vi "NAI8810A.vi"(8 "error in":errorcluster) -> (0 "error out":errorcluster)   [LabVIEW 2020]
uses:
  SubVIs/NAI8810A_TypeDefs.llb/AngleDifferenceButton.ctl
  <vilib>/Utility/miscctls.llb/LVPointTypeDef.ctl
  LabVIEW 2020 Toolkits/toolkits_lv2020_32bit/Synchronization.llb/SynchRefs_SetGet.ctl
  SubVIs/NAI8810A_TypeDefs.llb/NAI8810A_Command.ctl
  LabVIEW 2020 Toolkits/VI Server Toolkit/VI Server Libraries/VI Server_GetControl.llb/VI Server_STR_Get.vi
  <vilib>/Utility/inputDevices.llb/closeKeyboard.vi
  LabVIEW 2020 Toolkits/VI Server Toolkit/VI Server Toolkit LV2013.lvlib
panel:
  out "System.Message":string
  in  "UDP.Setup":bool
  in  "Help":bool
  in  "FP.Hide":bool caption="FrontPanel.Hide"
  in  "EXIT":bool
  in  "Tab.Main":T1(tab)
  in  "Ch1.Hold":bool
  in  "Tab.Ch1.Help":bool
  in  "Tab.Ch1.SetUp":bool
  in  "Tab.Ch1.IntRef":bool
  in  "Tab.Ch1.DualCh":bool
  in  "Tab.Ch1.Ch2":bool
  in  "Tab.Ch1.Ch1":bool
  out "Ch1.Degree":dbl caption="Degree" format="%0.4f"
  in  "Ch1.Input.Front/Rear":bool
  in  "Ch1.Local/Remote":bool
  in  "Ch1.Ratio":bool
  in  "Ch1.Graph":bool
  in  "Ch1.AnalogDisplay":bool
  in  "Ch1.EnableAngleOffsetCalc":bool
  in  "Ch1.TestAngleReadings":bool
  in  "Ch1.Ave.AnglesReadings":bool
  in  "Ch1.SYN/RSL":bool
  in  "Ch1.Internal/External.Ref":bool
  out "Ch1.Velocity":dbl format="%0.1f dps"
  out "Ch1.Frequency":dbl format="%0.2f Hz"
  out "Ch1.Line-to-Line.Voltage":dbl format="%0.2f mV"
  out "Ch1.Ref.Voltage":dbl format="%0.2f mV"
  in  "Ch2.Ave.AnglesReadings":bool
  in  "Ch2.Input.Front/Rear":bool
  out "Ch2.Line-to-Line.Voltage":dbl format="%0.2f mV"
  in  "Ch2.Hold":bool
  in  "Ch2.Graph":bool
  in  "Ch2.SYN/RSL":bool
  in  "Ch2.Internal/External.Ref":bool
  in  "Ch2.EnableAngleOffsetCalc":bool
  in  "Ch2.TestAngleReadings":bool
  in  "Ch2.Ratio":bool
  in  "Ch2.Local/Remote":bool
  out "Ch2.Velocity":dbl format="%0.1f dps"
  out "Ch2.Ref.Voltage":dbl format="%0.2f mV"
  out "Ch2.Degree":dbl caption="Degree" format="%0.4f"
  in  "Tab.Ch2.Ch2":bool
  in  "Tab.Ch2.Ch1":bool
  in  "Tab.Ch2.DualCh":bool
  in  "Tab.Ch2.IntRef":bool
  in  "Tab.Ch2.SetUp":bool
  in  "Tab.Ch2.Help":bool
  out "Ch2.Frequency":dbl format="%0.2f Hz"
  in  "Ch2.AnalogDisplay":bool
  in  "Ch1-2.Local/Remote":bool
  in  "Ch1-2.Ch2.AngleDifference":T2
  out "Ch1-2.Ch2.Frequency":dbl format="%0.2f Hz"
  out "Ch1-2.Ch2.Line-to-Line.Voltage":dbl format="%0.2f mV"
  out "Ch1-2.Ch2.Ref.Voltage":dbl format="%0.2f mV"
  in  "Ch1-2.Ch2.Ave.AnglesReadings":bool
  in  "Ch1-2.Ch2.Hold":bool
  in  "Ch1-2.Ch2.SYN/RSL":bool
  in  "Ch1-2.Ch2.Internal/External.Ref":bool
  out "Ch1-2.Ch2.Degree":dbl caption="Degree" format="%0.4f"
  in  "Ch1-2.Ch1.TestAngleReadings":bool
  in  "Ch1-2.Ch1.Ave.AnglesReadings":bool
  out "Ch1-2.Ch1.Line-to-Line.Voltage":dbl format="%0.2f mV"
  out "Ch1-2.Ch1.Ref.Voltage":dbl format="%0.2f mV"
  out "Ch1-2.Ch1.Frequency":dbl format="%0.2f Hz"
  in  "Ch1-2.Graph":bool
  in  "Ch1-2.Ratio":bool
  in  "Ch1-2.Input.Front/Rear":bool
  in  "Ch1-2.Ch1.SYN/RSL":bool
  in  "Ch1-2.Ch1.Internal/External.Ref":bool
  in  "Ch1-2.Ch1.Hold":bool
  out "Ch1-2.Ch1.Degree":dbl caption="Degree" format="%0.4f"
  in  "Tab.Ch1-2.SetUp":bool
  in  "Tab.Ch1-2.IntRef":bool
  in  "Tab.Ch1-2.Ch2":bool
  in  "Tab.Ch1-2.Ch1":bool
  in  "Tab.Ch1-2.Ch1-2":bool
  in  "Tab.Ch1-2.Help":bool
  in  "Ch1-2.Ch2.TestAngleReadings":bool
  in  "InternalRef.Frequency.Increment":bool
  in  "InternalRef.Input.Front/Rear":bool
  in  "InternalRef.Delta":u16=1 min=1 max=20000
  in  "InternalRef.115V":bool
  in  "InternalRef.26V":bool
  in  "InternalRef.Signal.Out":u16(ring) items=["AVAILABLE", "NOT AVAILABLE"]
  in  "InternalRef.Local/Remote":bool
  in  "InternalRef.Ratio":bool
  in  "InternalRef.Graph":bool
  in  "InternalRef.Frequency":dbl=47.0 caption="Degree" min=47.0 max=20000.0 step=0.1 format="%0.2f"
  in  "InternalRef.Voltage":dbl=2.0 caption="Degree" min=2.0 max=115.0 step=0.1 format="%0.1f"
  in  "Tab.IntRef.Help":bool
  in  "Tab.IntRef.IntRef":bool
  in  "Tab.IntRef.Ch1":bool
  in  "Tab.IntRef.Ch2":bool
  in  "Tab.IntRef.Ch1-2":bool
  in  "Tab.IntRef.SetUp":bool
  in  "AutomaticUpdate":bool caption="Automatic Update"
  in  "TCP/IP.Setup":bool
  in  "Ch2.Bandwidth.Value":u16=6 caption="Bandwidth Value (6-1200 Hz)" min=6 max=1200 format="%d Hz"
  in  "Ch2.AutoBandwidth":bool caption="Auto-Bandwidth"
  in  "Ch1.Bandwidth.Value":u16=6 caption="Bandwidth Value (6-1200 Hz)" min=6 max=1200 format="%d Hz"
  in  "Ch1.AutoBandwidth":bool caption="Auto-Bandwidth"
  in  "AngleResolution":u16(ring) caption="Angle Res:" items=["0", "1", "2", "3", "4"]
  in  "AngleDisplay.Format":u16(ring) caption="Angle Display:" items=["360", "180", "MIN"]
  in  "Setup.DONE":bool
  in  "UpdateTime.Ref.Parameters":u32=5 caption="Ref. Data" min=5 max=20000 format="%d msec"
  in  "UpdateTime.Degrees":u32=5 caption="Degrees" min=5 max=20000 format="%d msec"
  out "UDP.Responce.String":string caption="UDP: Responce String"
  in  "UDP.Responce.String.Monitor":bool
  in  "UDP.Test.String2.Send":bool
  in  "UDP.Test.String2":string caption="UDP: Test String 2"
  in  "UDP.IP.Address":string caption="UDP: IP Address"
  in  "UDP.LocalPort.Write":u16 caption="UDP: Local Port.Write"
  in  "UDP.Port.RT":u16 caption="UDP: Port.RT"
  in  "UDP.Port.BC":u16 caption="UDP: Port.BC"
  in  "UDP.Test.String1":string caption="UDP: Test String 1"
  in  "UDP.Test.String1.Send":bool
  in  "AveAnglesReadings.DONE":bool
  in  "Ch2.AveragingInterval":u16=10 caption="Averaging Interval" min=10 max=10000 format="%d msec"
  in  "Ch2.AverageAnglesReadings":bool caption="Ch2: Average Angles Readings"
  in  "Ch1.AveragingInterval":u16=10 caption="Averaging Interval" min=10 max=10000 format="%d msec"
  in  "Ch1.AverageAnglesReadings":bool caption="Ch1: Average Angles Readings"
  in  "Ch2.TestAngleReading.Step":dbl=0.0001 caption="Angle Step" min=0.0001 max=359.9999 format="%0.4f deg"
  in  "Ch2.TestAngleReading.Limit.LO":dbl caption="Angle Limit LO" min=0.0 max=359.9999 format="%0.4f deg"
  in  "Ch2.TestAngleReading.Limit.HI":dbl caption="Angle Limit HI" min=0.0 max=359.9999 format="%0.4f deg"
  in  "Ch2.TestAngleReading.Comparision.Mode":bool caption="Ch1.TestAngleReading"
  in  "Ch2.TestAngleReading.ENBL":bool caption="Ch1.TestAngleReading"
  in  "Ch1.TestAngleReading.Step":dbl=0.0001 caption="Angle Step" min=0.0001 max=359.9999 format="%0.4f deg"
  in  "Ch1.TestAngleReading.Limit.LO":dbl caption="Angle Limit LO" min=0.0 max=359.9999 format="%0.4f deg"
  in  "Ch1.TestAngleReading.Limit.HI":dbl caption="Angle Limit HI" min=0.0 max=359.9999 format="%0.4f deg"
  in  "Ch1.TestAngleReading.Comparision.Mode":bool caption="Ch1.TestAngleReading"
  in  "Ch1.TestAngleReading.ENBL":bool caption="Ch1.TestAngleReading"
  in  "TestAnglesReadings.DONE":bool
  in  "Ratio.Value":u8=2 caption="Ratio                              : 1" min=1
  in  "Ratio.Mode":bool
  in  "Ratio.DONE":bool
  in  "Chart.Config.ClearBuffer":bool
  in  "Chart.Config":bool
  in  "Chart.Start":bool
  in  "Chart.DONE":bool
  out "Chart":dbl(graph)
  in  "Chart.Config.SamplingRate.Units":u16(ring) items=["msec", "sec", "min"]
  in  "Chart.Config.SamplingRate":u16 caption="Sampling Rate"
  in  "Chart.Config.DataToPlot":u16(ring) caption="Data To Plot" items=["Angle", "Angl Error", "Velocity"]
  in  "Chart.Config.ChannelSelection":u16(ring) caption="Chan Display" items=["BOTH", "CH1", "CH2"]
  in  "Chart.Config.DataToPlot.Step":dbl=0.0001 caption="Angle Step" min=0.0001 max=359.9999 format="%0.4f deg"
  in  "GraphConfig.DONE":bool
  in  "MonitorCommandExecution":bool caption="Monitor Command Execution"
  in  "TCP/IP.Command.Send":bool
  out "TCP/IP.InstrumentResponce":string caption="Instrument Responce"
  in  "TCP/IP.Command":string="*IDN?" caption="Command"
  in  "TCP/IP.Instrument.ID":string="NORTH ATLANTIC,5330A-10" caption="TCP/IP: Instrument ID"
  in  "TCP/IP.Port":u16=23 caption="TCP/IP: Port"
  in  "TCP/IP.Address":string="192.168.4.5" caption="TCP/IP: Address"
  in  "TCP/IP.DONE":bool
  # "Options: Current Configuration"
  # "Options: Bandwidth"
  # "Channel 2"
  # "Channel 1"
  # "Update Time"
  # "Chanel 2"
  # "Chanel 1"
  # "Ratio"
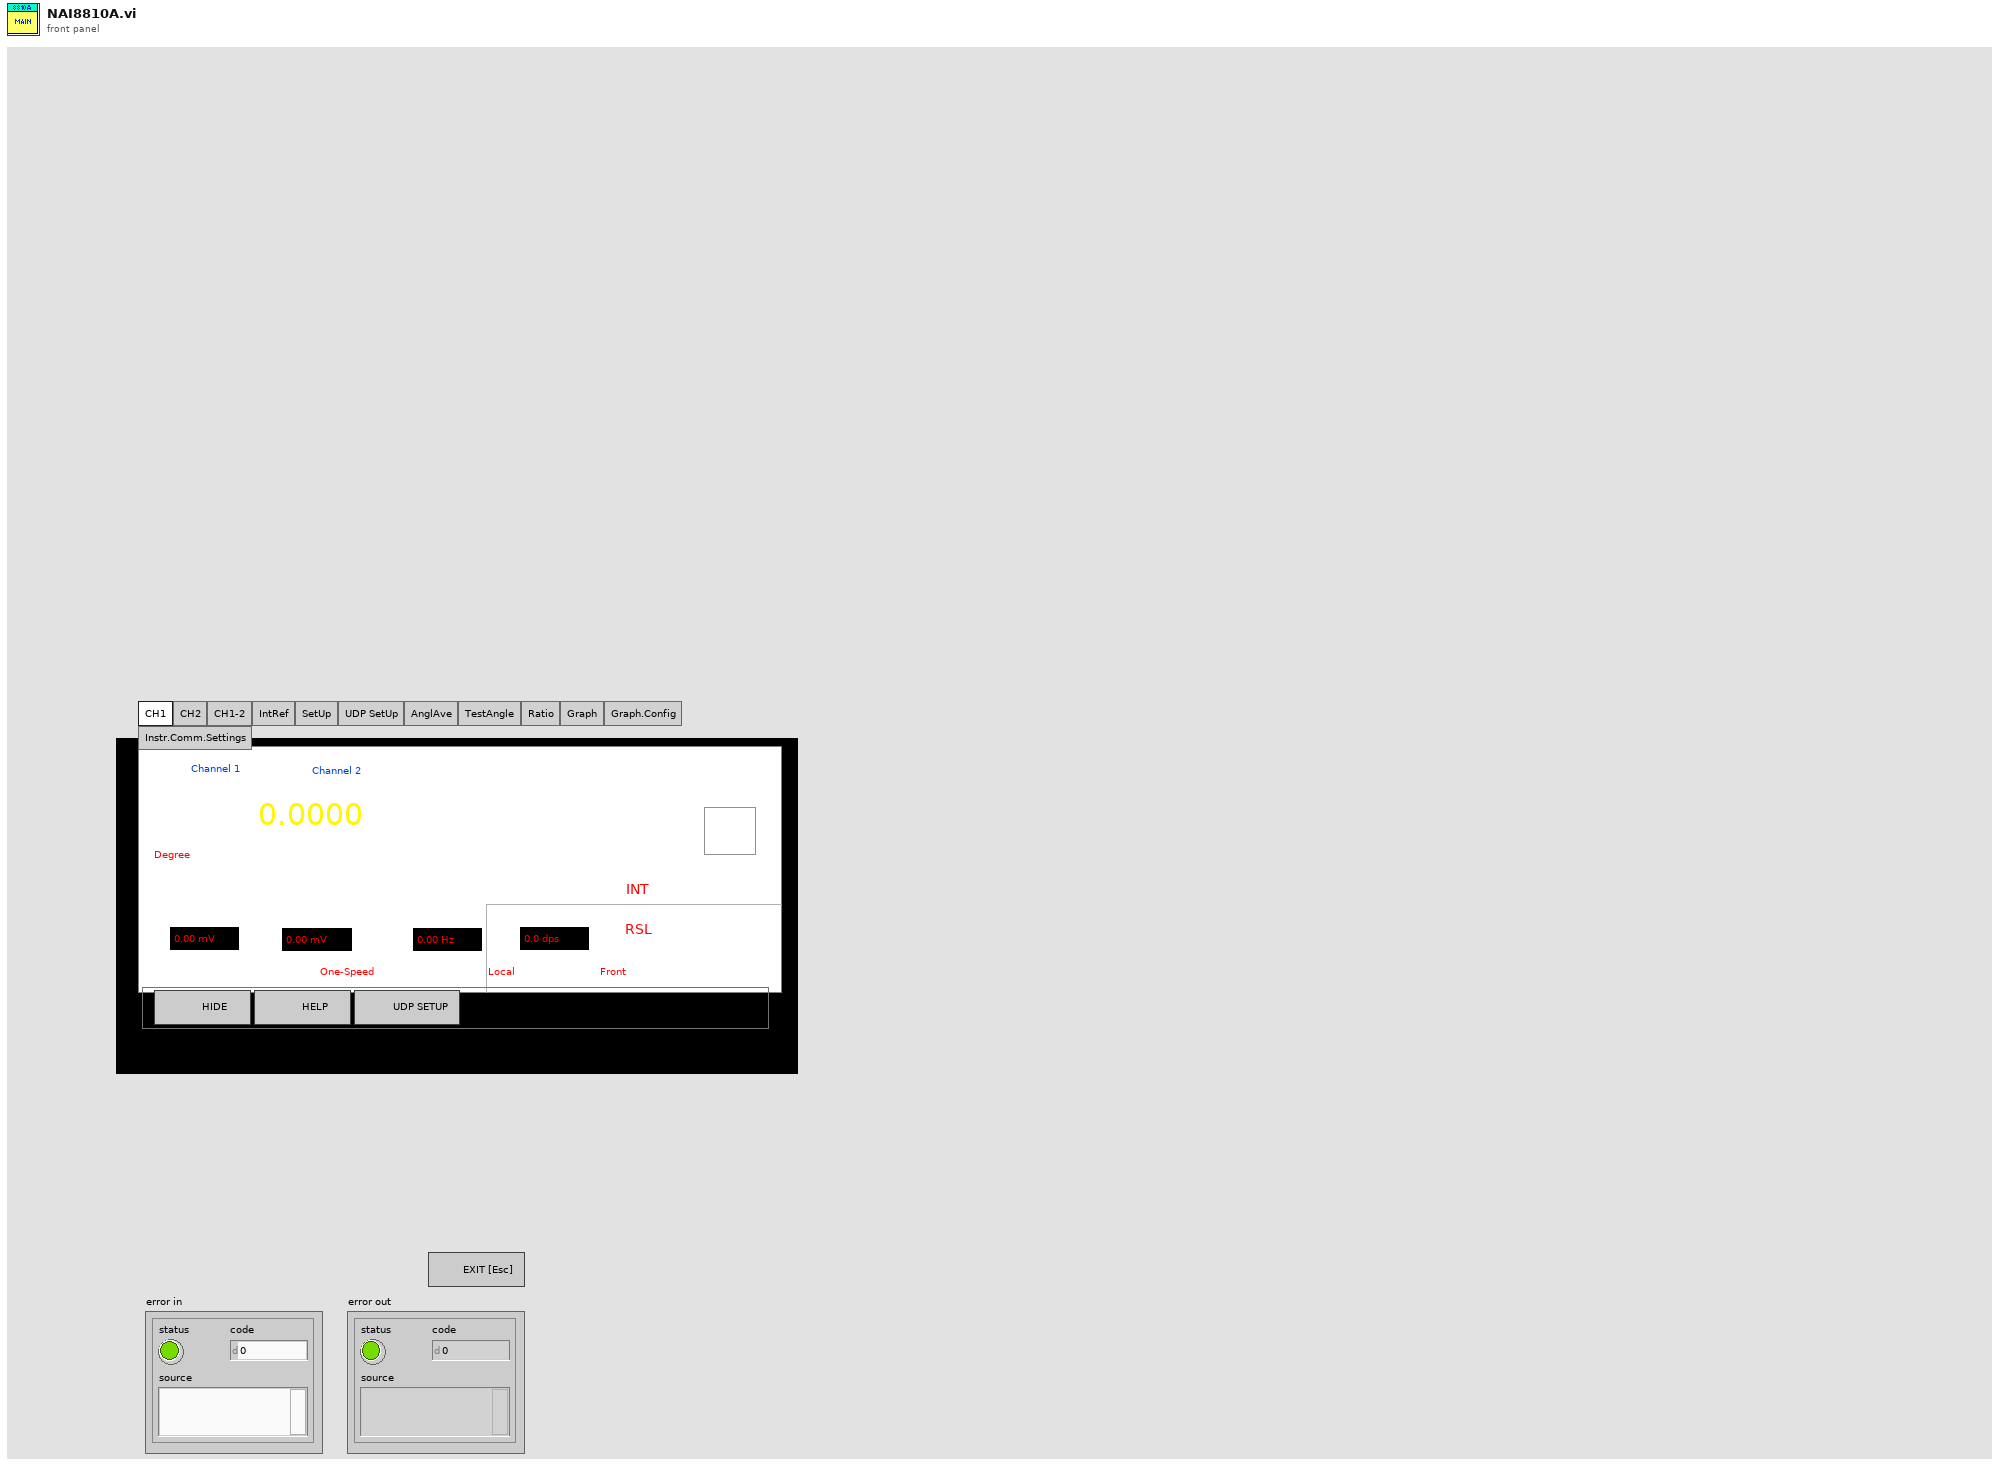
[diagram p1: front panel]
types:
  T1 = enum32{"CH1", "CH2", "CH1-2", "IntRef", "SetUp", "UDP SetUp", "AnglAve", "TestAngle", "Ratio", "Graph", "Graph.Config", "Instr.Comm.Settings"}
  T2 = typedef "AngleDifferenceButton.ctl" = bool
  T3 = typedef "LVPointTypeDef.ctl" = cluster{"Horizontal":i16, "Vertical":i16}
  T4 = typedef "VI Server_RefsCluster.ctl" = cluster{"Labels":string[], "Refs":refnum<vi>[], "VI Ref":refnum<vi>}
  T5 = typedef "SynchRefs_SetGet.ctl" = enum16{"Set", "Get"}
  T6 = typedef "NAI8810A_Command.ctl" = enum16{"", "*IDN?", "Reference Mode", "Signal Mode", "Channel 1 Input Connector", "Track/Latch Angle", "Reference Generator Voltage", "Reference Generator Frequency", "Reference Generator Output State", "Reference Generator Overcurrent State", "Reference Generator Overcurrent State RST ", "Angle Difference", "Angle Difference Get", "Angle Ch1", "Reference Voltage", "Angle Ch2", "Angle Ch1-2", "Angle Averaging ON/OFF", "Ch1.Angle Averaged", "Ch2.Angle Averaged", "Angle.AverageRate", "Ch1.Velocity", "Ch2.Velocity", "Ch1.Line-to-Line Voltage", "Ch2.Line-to-Line Voltage", "Ch1.ReferenceVoltage", "Ch2.ReferenceVoltage", "Ch1.ReferenceFrequency", "Ch2.ReferenceFrequency", "LOCAL/REMOTE", "ANG_LIMIT.ON|OFF", "ANG_LIMIT.CMP.ABS|ERR", "ANG_LIMIT.HI", "ANG_LIMIT.LO", "ANG_LIMIT.STEP", "Ratio", "AngleDisplay.Format", "Angles.Resolution", "Bandwidth.AUTO", "Bandwidth.SET", "Plot.ChannelSelection", "Data-to-Plot", "Buffering: SampleRate", "Clear Buffer", "Buffer: Record"}
  T7 = enum32{"CH1", "CH2", "CH1-2", "IntRef", "SetUp", "UDP SetUp", "AnglAve", "TestAngle"}
  T8 = enum32{"CH1", "CH2", "CH1-2", "IntRef", "SetUp", "UDP SetUp", "AnglAve", "TestAngle", "Ratio", "Graph", "Graph.Config"}
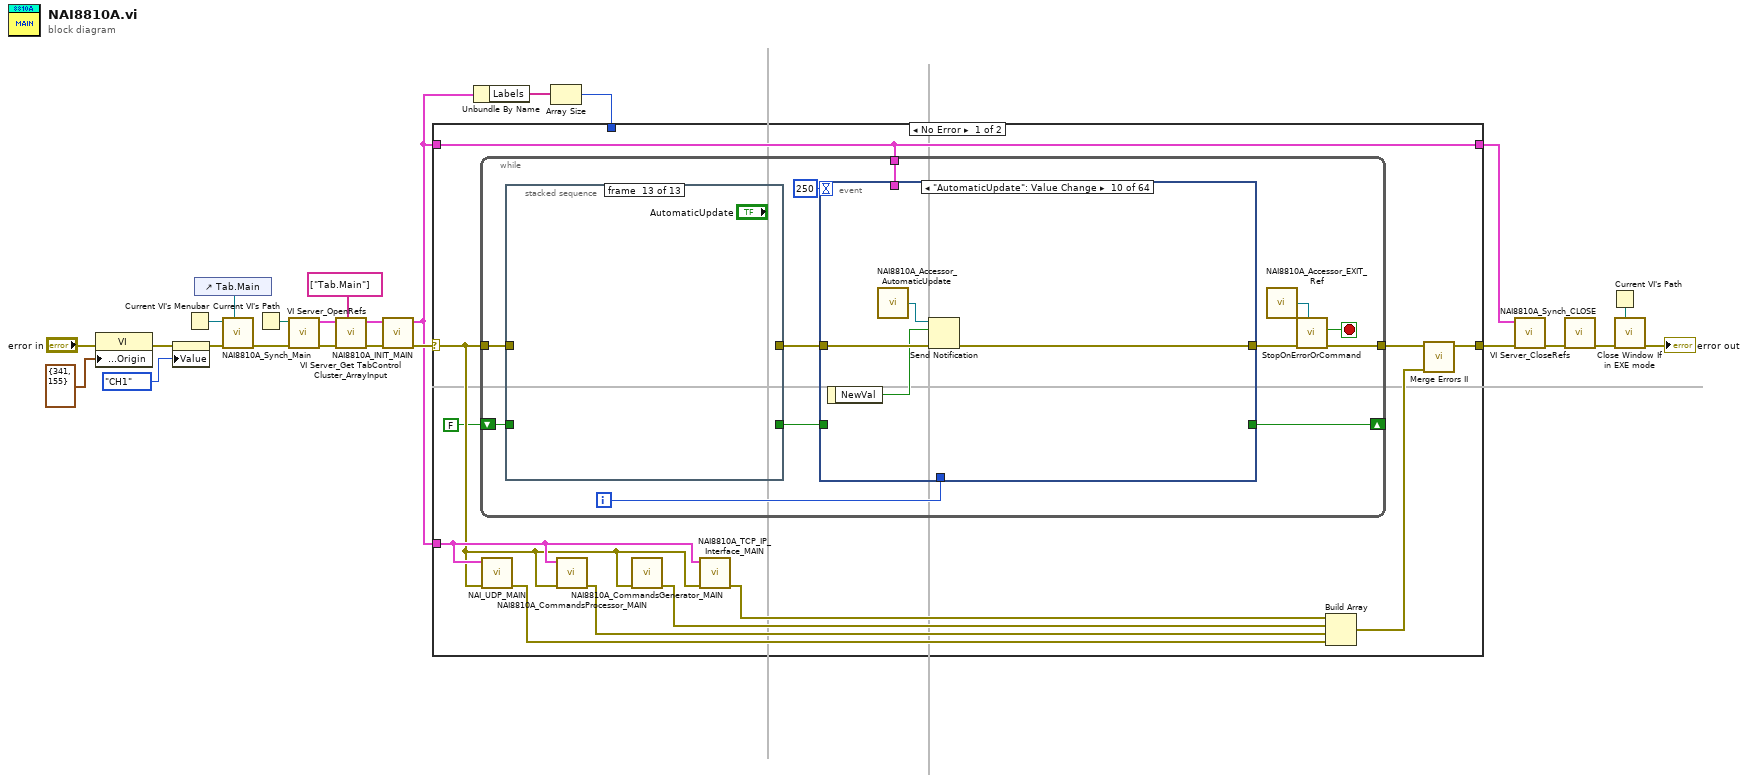
[diagram p0: block diagram]
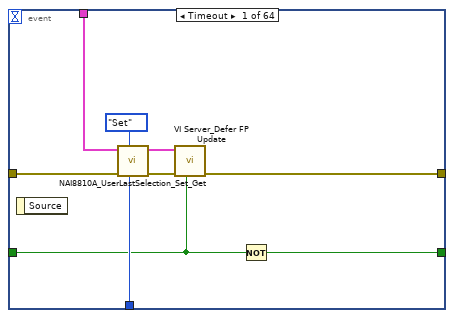
[diagram p2: hidden frame]
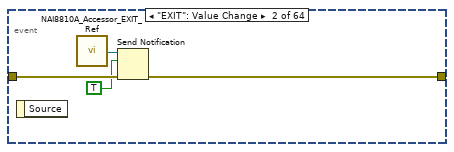
[diagram p3: hidden frame]
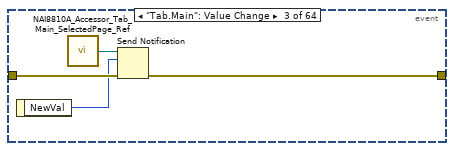
[diagram p4: hidden frame]
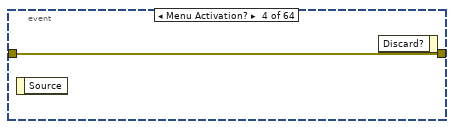
[diagram p5: hidden frame]
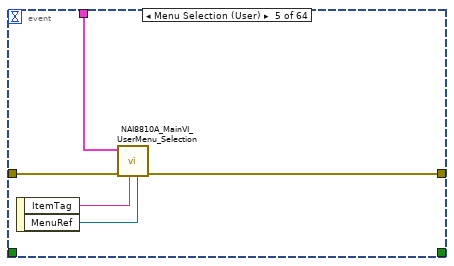
[diagram p6: hidden frame]
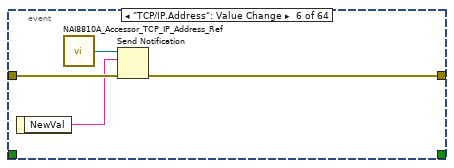
[diagram p7: hidden frame]
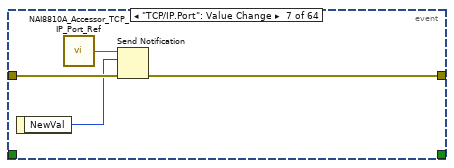
[diagram p8: hidden frame]
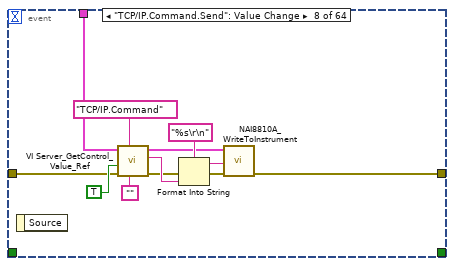
[diagram p9: hidden frame]
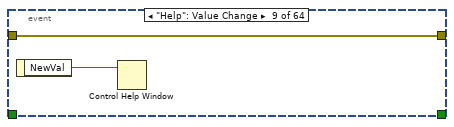
[diagram p10: hidden frame]
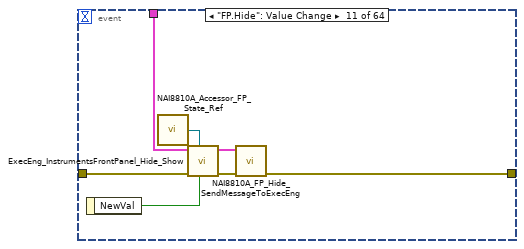
[diagram p11: hidden frame]
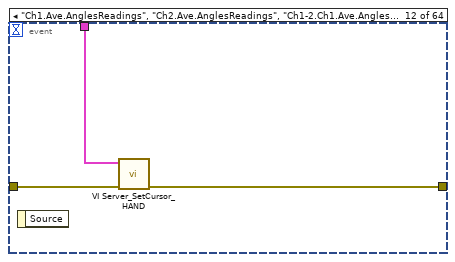
[diagram p12: hidden frame]
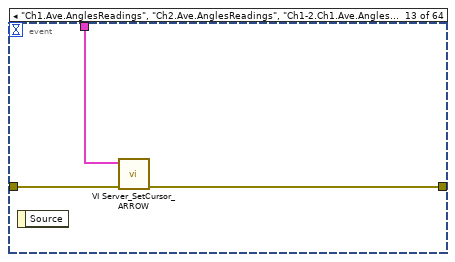
[diagram p13: hidden frame]
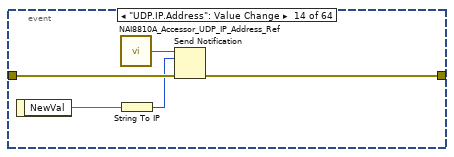
[diagram p14: hidden frame]
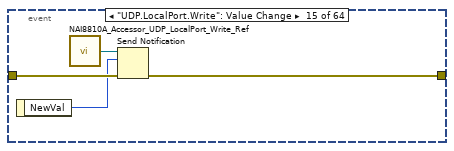
[diagram p15: hidden frame]
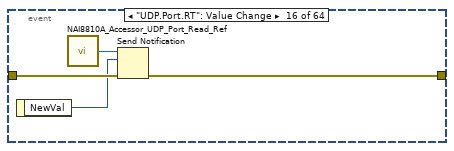
[diagram p16: hidden frame]
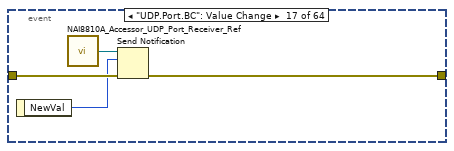
[diagram p17: hidden frame]
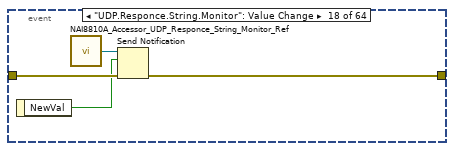
[diagram p18: hidden frame]
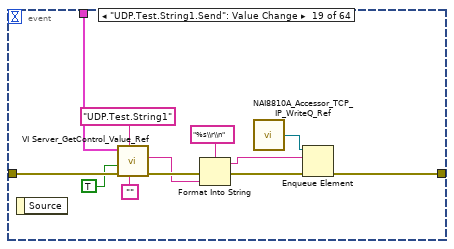
[diagram p19: hidden frame]
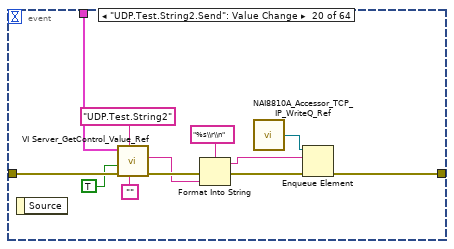
[diagram p20: hidden frame]
diagram:
  n1 = property class="VI"(error in="error in", "Front Panel Window:Origin"=T3 {"Horizontal"=341, "Vertical"=155}) -> (error out=w3:errorcluster)  [unwired: 1 in, 1 out]
  n2 = property on="Tab.Main" class="TabCtl (strict)"(error in=w3, "Value"=T1."CH1" ("Tab.Main")) -> (error out=w2:errorcluster)  [unwired: 1 in, 1 out]
  n3 = Current VI's Menubar() -> (w7:refnum<k9>)
  n4 = control-ref of="Tab.Main"() -> (w11:refnum<vi>)
  n5 = call "NAI8810A_Synch_Main.vi"("Tab.Main.Ref"=w11, "error in"=w2, "menu reference"=w7) -> ("error out"=w14:errorcluster)  [unwired: 8 in]
  n6 = Current VI's Path() -> (path=w21:path)
  n7 = call "VI Server_OpenRefs.vi"("error in"=w14, "VI Path"=w21) -> ("error out"=w24:errorcluster, "VI Server.RefsCluster"=w23:T4)  [unwired: 8 in]
  n8 = call "VI Server_Get TabControl Cluster_ArrayInput.vi"("TabControl Labels[]"=string[] ["Tab.Main"], "error in"=w24, "VI Server Cluster"=w23) -> ("error out"=w16:errorcluster, "VI Server Cluster.OUT"=w15:T4)  [unwired: 7 in]
  n9 = call "NAI8810A_INIT_MAIN.vi"("error in (no error)"=w16, "VI Server Cluster"=w15) -> ("error out"=w17:errorcluster, "VI Server Cluster DUP"=w10:T4)  [unwired: 8 in]
  n10 = Unbundle By Name(w10) -> ("Labels"=w9:string[])
  n11 = Array Size(array=w9) -> (size(s)=w8:i32)
  n12 = case shown="No Error" w17 {
    selector: w17 -> [w27 w434]
    tunnel: [w34 w434] -> w20
    tunnel: w10 -> [w28 _]
    tunnel: w10 -> [w31 w433]
    tunnel: [w31 w433] -> w18
    tunnel: w8 -> [_ _]
    frame No Error {
      n13 = while {
        tunnel: w27 -> [w47]
        tunnel: [w44] -> w35
        tunnel: w31 -> [w40]
        shift-right: [w36] -> _
        shift-left: FALSE -> [w38]
        i -> [w39]
        stop <- w42 stop-if-true
        n14 = stacked-sequence {
          tunnel: w47 -> [w431 _ _ _ _ _ _ _ _ _ _ _ _]
          tunnel: [w431 _ _ _ _ _ _ _ _ _ _ _ _] -> w45
          tunnel: w38 -> [_ w432 _ _ _ _ _ _ _ _ _ _ _]
          tunnel: [_ w432 _ _ _ _ _ _ _ _ _ _ _] -> w37
          frame #0 {
          }
          frame #1 {
          }
          frame #2 {
          }
          frame #3 {
          }
          frame #4 {
          }
          frame #5 {
          }
          frame #6 {
          }
          frame #7 {
          }
          frame #8 {
          }
          frame #9 {
          }
          frame #10 {
          }
          frame #11 {
          }
          frame #12 {
          }
        }
        n15 = event shown="[9] \"AutomaticUpdate\": Value Change" {
          selector: _ -> [_ _ _ _ _ _ _ _ _ _ _ _ _ _ _ _ _ _ _ _ _ _ _ _ _ _ _ _ _ _ _ _ _ _ _ _ _ _ _ _ _ _ _ _ _ _ _ _ _ _ _ _ _ _ _ _ _ _ _ _ _ _ _ _]
          dyn-events: _ -> [_ _ _ _ _ _ _ _ _ _ _ _ _ _ _ _ _ _ _ _ _ _ _ _ _ _ _ _ _ _ _ _ _ _ _ _ _ _ _ _ _ _ _ _ _ _ _ _ _ _ _ _ _ _ _ _ _ _ _ _ _ _ _ _]
          timeout: 250 -> [_ _ _ _ _ _ _ _ _ _ _ _ _ _ _ _ _ _ _ _ _ _ _ _ _ _ _ _ _ _ _ _ _ _ _ _ _ _ _ _ _ _ _ _ _ _ _ _ _ _ _ _ _ _ _ _ _ _ _ _ _ _ _ _]
          tunnel: w45 -> [w56 w60 w64 w65 w70 w74 w78 w84 w92 w96 w103 w106 w109 w114 w118 w122 w126 w130 w142 w154 w158 w160 w168 w183 w198 w213 w225 w228 w231 w239 w251 w258 w260 w264 w267 w269 w272 w277 w285 w293 w304 w315 w326 w333 w335 w339 w343 w346 w350 w354 w358 w371 w384 w387 w392 w395 w402 w405 w411 w417 w420 w423 w424 w430]
          tunnel: [w48 w58 w62 w65 w68 w73 w75 w79 w92 w95 w98 w104 w107 w113 w117 w121 w125 w127 w141 w153 w155 w163 w178 w193 w204 w219 w224 w227 w230 w240 w252 w259 w261 w262 w266 w268 w271 w278 w284 w289 w298 w309 w320 w332 w336 w337 w341 w344 w349 w353 w357 w363 w376 w388 w390 w394 w401 w407 w410 w415 w418 w421 w425 w429] -> w43
          tunnel: w40 -> [w55 _ _ _ w69 _ _ w82 _ _ w101 w105 w108 _ _ _ _ _ w140 w152 _ w159 _ _ _ _ _ w226 w229 _ _ w257 _ _ _ _ _ _ w283 w286 w297 w308 w319 w331 w334 w338 _ w345 w348 _ _ w370 w383 w386 w391 _ w400 _ _ w416 w419 w422 w426 w428]
          tunnel: w39 -> [w53 _ _ _ _ _ _ _ _ _ _ _ _ _ _ _ _ _ _ _ _ _ _ _ _ _ _ _ _ _ _ _ _ _ _ _ _ _ _ _ _ _ _ _ _ _ _ _ _ _ _ _ _ _ _ _ _ _ _ _ _ _ _ _]
          tunnel: w37 -> [w49 _ _ _ _ _ _ _ _ _ _ _ _ _ _ _ _ _ _ _ _ _ _ _ _ _ _ _ _ _ _ _ _ _ _ _ _ _ _ _ _ _ _ _ _ _ _ _ _ _ _ _ _ _ _ _ _ _ _ _ _ _ _ _]
          tunnel: [w52 _ _ _ _ _ _ _ _ _ _ _ _ _ _ _ _ _ _ _ _ _ _ _ _ _ _ _ _ _ _ _ _ _ _ _ _ _ _ _ _ _ _ _ _ _ _ _ _ _ _ _ _ _ _ _ _ _ _ _ _ _ _ _] -> w36
          event Timeout {
            n16 = event-data() -> ()  [unwired: 1 in, 1 out]
            n17 = call "NAI8810A_UserLastSelection_Set_Get.vi"("LoopCounter"=w53, "SynchRefs.Set/Get"=SynchRefs_SetGet."Set", "error in"=w56, "VI Server.RefsCluster"=w55) -> ("error out"=w51:errorcluster, "VI Server.RefsCluster.DUP"=w50:T4)  [unwired: 6 in]
            n18 = call "VI Server_Defer FP Update.vi"("Defer Panel Updates? (F)"=w49, "error in"=w51, "VI Server Cluster"=w50) -> ("error out"=w48:errorcluster)  [unwired: 7 in, 1 out]
            n19 = Not(x=w49) -> (.not. x?=w52:bool)
          }
          event "EXIT": Value Change {
            n20 = event-data() -> ()  [unwired: 1 in, 1 out]
            n21 = call "NAI8810A_Accessor_EXIT_Ref.vi"() -> ("EXIT"=w59:refnum<notifier>)  [unwired: 6 in]
            n22 = Send Notification(notification=TRUE, notifier=w59, error in (no error)=w60) -> (error out=w58:errorcluster)  [unwired: 1 out]
          }
          event "Tab.Main": Value Change {
            n23 = event-data() -> ("NewVal"=w61:T1)  [unwired: 1 in]
            n24 = call "NAI8810A_Accessor_Tab_Main_SelectedPage_Ref.vi"() -> ("Tab.Main.SelectedPage"=w63:refnum<notifier>)  [unwired: 6 in]
            n25 = Send Notification(notification=w61, notifier=w63, error in (no error)=w64) -> (error out=w62:errorcluster)  [unwired: 1 out]
          }
          event Menu Activation? {
            n26 = event-data() -> ()  [unwired: 1 in, 1 out]
            n27 = event-data() -> ()  [unwired: 2 in, 1 out]
          }
          event Menu Selection (User) {
            n28 = event-data() -> ("ItemTag"=w67:string, "MenuRef"=w66:refnum<k9>)  [unwired: 1 in]
            n29 = call "NAI8810A_MainVI_UserMenu_Selection.vi"("MenuRef"=w66, "Menu.ItemTag"=w67, "error in"=w70, "VI Server.RefsCluster"=w69) -> ("error out"=w68:errorcluster)  [unwired: 6 in, 1 out]
          }
          event "TCP/IP.Address": Value Change {
            n30 = event-data() -> ("NewVal"=w71:string)  [unwired: 1 in]
            n31 = call "NAI8810A_Accessor_TCP_IP_Address_Ref.vi"() -> ("TCP/IP.Address"=w72:refnum<notifier>)  [unwired: 6 in]
            n32 = Send Notification(notification=w71, notifier=w72, error in (no error)=w74) -> (error out=w73:errorcluster)  [unwired: 1 out]
          }
          event "TCP/IP.Port": Value Change {
            n33 = event-data() -> ("NewVal"=w76:u16)  [unwired: 1 in]
            n34 = call "NAI8810A_Accessor_TCP_IP_Port_Ref.vi"() -> ("TCP/IP.Port"=w77:refnum<notifier>)  [unwired: 6 in]
            n35 = Send Notification(notification=w76, notifier=w77, error in (no error)=w78) -> (error out=w75:errorcluster)  [unwired: 1 out]
          }
          event "TCP/IP.Command.Send": Value Change {
            n36 = event-data() -> ()  [unwired: 1 in, 1 out]
            n37 = call-poly "VI Server_GetControl_Value_Ref.vi"("DataType"="", "Control.Label"="TCP/IP.Command", "error in"=w84, "SingleInstance"=TRUE, "VI Server.RefsCluster"=w82) -> ("error out"=w89:errorcluster, "Value"=w90:string, "VI Server.RefsCluster.DUP"=w81:T4)  [unwired: 3 in, 1 out]
            n38 = Format Into String(format string="%s\r\n", error in=w89, w90) -> (resulting string=w80:string, error out=w83:errorcluster)  [unwired: 1 in]
            n39 = call "NAI8810A_WriteToInstrument.vi"("error in"=w83, "Command"=w80, "VI Server.RefsCluster"=w81) -> ("error out"=w79:errorcluster)  [unwired: 7 in, 1 out]
          }
          event "Help": Value Change {
            n40 = event-data() -> ("NewVal"=w91:bool)  [unwired: 1 in]
            n41 = Control Help Window(1:w91) -> ()  [unwired: 1 in]
          }
          event "AutomaticUpdate": Value Change {
            n42 = event-data() -> ("NewVal"=w93:bool)  [unwired: 1 in]
            n43 = call "NAI8810A_Accessor_AutomaticUpdate.vi"() -> ("AutomaticUpdate"=w94:refnum<notifier>)  [unwired: 6 in]
            n44 = Send Notification(notification=w93, notifier=w94, error in (no error)=w96) -> (error out=w95:errorcluster)  [unwired: 1 out]
          }
          event "FP.Hide": Value Change {
            n45 = event-data() -> ("NewVal"=w102:bool)  [unwired: 1 in]
            n46 = call "NAI8810A_Accessor_FP_State_Ref.vi"() -> ("FP.State"=w100:refnum<notifier>)  [unwired: 6 in]
            n47 = call "ExecEng_InstrumentsFrontPanel_Hide_Show.vi"("FP.Hide/Show"=w102, "FP.State"=w100, "error in (no error)"=w103, "VI Server Cluster"=w101) -> ("error out"=w99:errorcluster, "VI Server Cluster DUP"=w97:T4)  [unwired: 6 in]
            n48 = call "NAI8810A_FP_Hide_SendMessageToExecEng.vi"("error in (no error)"=w99, "VI Server Cluster"=w97) -> ("error out"=w98:errorcluster)  [unwired: 9 in]
          }
          event "Ch1.Ave.AnglesReadings", "Ch2.Ave.AnglesReadings", "Ch1-2.Ch1.Ave.AnglesReadings", "Ch1-2.Ch2.Ave.AnglesReadings", "Ch1.TestAngleReadings", "Ch2.TestAngleReadings", "Ch1-2.Ch1.TestAngleReadings", "Ch1-2.Ch2.TestAngleReadings", "Ch1.EnableAngleOffsetCalc", "Ch2.EnableAngleOffsetCalc", "Ch1.Graph", "Ch2.Graph", "Ch1-2.Graph", "InternalRef.Graph", "Tab.Ch1.Ch1", "Tab.Ch1.Ch2", "Tab.Ch1.DualCh", "Tab.Ch1.IntRef", "Tab.Ch1.SetUp", "Tab.Ch1.Help", "Tab.Ch2.Help", "Tab.Ch2.SetUp", "Tab.Ch2.IntRef", "Tab.Ch2.DualCh", "Tab.Ch2.Ch1", "Tab.Ch2.Ch2", "Tab.Ch1-2.SetUp", "Tab.Ch1-2.IntRef", "Tab.Ch1-2.Ch2", "Tab.Ch1-2.Ch1", "Tab.Ch1-2.Ch1-2", "Tab.Ch1-2.Help", "Tab.IntRef.SetUp", "Tab.IntRef.Ch1-2", "Tab.IntRef.Ch2", "Tab.IntRef.Ch1", "Tab.IntRef.IntRef", "Tab.IntRef.Help", "Ch1.Ratio", "Ch2.Ratio", "Ch1-2.Ratio", "InternalRef.Ratio", "Ch1.Local/Remote", "Ch2.Local/Remote", "Ch1-2.Local/Remote", "InternalRef.Local/Remote", "Ch1.Input.Front/Rear", "Ch2.Input.Front/Rear", "Ch1-2.Input.Front/Rear", "InternalRef.Input.Front/Rear", "Ch1.Hold", "Ch2.Hold", "Ch1-2.Ch1.Hold", "Ch1-2.Ch2.Hold", "Ch1.Internal/External.Ref", "Ch2.Internal/External.Ref", "Ch1-2.Ch1.Internal/External.Ref", "Ch1-2.Ch2.Internal/External.Ref", "Ch1.SYN/RSL", "Ch2.SYN/RSL", "Ch1-2.Ch1.SYN/RSL", "Ch1-2.Ch2.SYN/RSL", "FP.Hide", "UDP.Setup", "EXIT", "AveAnglesReadings.DONE", "TestAnglesReadings.DONE", "Ratio.DONE", "Chart.DONE", "Setup.DONE", "GraphConfig.DONE", "TCP/IP.DONE", "Ch1.AutoBandwidth", "Ch2.AutoBandwidth", "InternalRef.26V", "InternalRef.115V", "InternalRef.Signal.Out", "Ch1.AverageAnglesReadings", "Ch2.AverageAnglesReadings", "Chart.Start", "Chart.Config.ChannelSelection", "Chart.Config", "Chart.Config.DataToPlot", "Chart.Config.ClearBuffer", "Chart.Config.SamplingRate.Units", "Ratio.Mode", "InternalRef.Frequency.Increment": Mouse Enter {
            n49 = event-data() -> ()  [unwired: 1 in, 1 out]
            n50 = call "VI Server_SetCursor_HAND.vi"("error in"=w106, "VI Server.RefsCluster"=w105) -> ("error out"=w104:errorcluster)  [unwired: 8 in, 1 out]
          }
          event "Ch1.Ave.AnglesReadings", "Ch2.Ave.AnglesReadings", "Ch1-2.Ch1.Ave.AnglesReadings", "Ch1-2.Ch2.Ave.AnglesReadings", "Ch1.TestAngleReadings", "Ch2.TestAngleReadings", "Ch1-2.Ch1.TestAngleReadings", "Ch1-2.Ch2.TestAngleReadings", "Ch1.EnableAngleOffsetCalc", "Ch2.EnableAngleOffsetCalc", "Ch1.Graph", "Ch2.Graph", "Ch1-2.Graph", "InternalRef.Graph", "Tab.Ch1.Ch1", "Tab.Ch1.Ch2", "Tab.Ch1.DualCh", "Tab.Ch1.IntRef", "Tab.Ch1.SetUp", "Tab.Ch1.Help", "Tab.Ch2.Help", "Tab.Ch2.SetUp", "Tab.Ch2.IntRef", "Tab.Ch2.DualCh", "Tab.Ch2.Ch1", "Tab.Ch2.Ch2", "Tab.Ch1-2.SetUp", "Tab.Ch1-2.IntRef", "Tab.Ch1-2.Ch2", "Tab.Ch1-2.Ch1", "Tab.Ch1-2.Ch1-2", "Tab.Ch1-2.Help", "Tab.IntRef.SetUp", "Tab.IntRef.Ch1-2", "Tab.IntRef.Ch2", "Tab.IntRef.Ch1", "Tab.IntRef.IntRef", "Tab.IntRef.Help", "Ch1.Ratio", "Ch2.Ratio", "Ch1-2.Ratio", "InternalRef.Ratio", "Ch1.Local/Remote", "Ch2.Local/Remote", "Ch1-2.Local/Remote", "InternalRef.Local/Remote", "Ch1.Input.Front/Rear", "Ch2.Input.Front/Rear", "Ch1-2.Input.Front/Rear", "InternalRef.Input.Front/Rear", "Ch1.Hold", "Ch2.Hold", "Ch1-2.Ch1.Hold", "Ch1-2.Ch2.Hold", "Ch1.Internal/External.Ref", "Ch2.Internal/External.Ref", "Ch1-2.Ch1.Internal/External.Ref", "Ch1-2.Ch2.Internal/External.Ref", "Ch1.SYN/RSL", "Ch2.SYN/RSL", "Ch1-2.Ch1.SYN/RSL", "Ch1-2.Ch2.SYN/RSL", "FP.Hide", "UDP.Setup", "EXIT", "AveAnglesReadings.DONE", "TestAnglesReadings.DONE", "Ratio.DONE", "Chart.DONE", "Setup.DONE", "GraphConfig.DONE", "TCP/IP.DONE", "Ch1.AutoBandwidth", "Ch2.AutoBandwidth", "InternalRef.Signal.Out", "InternalRef.26V", "InternalRef.115V", "Ch1.AverageAnglesReadings", "Ch2.AverageAnglesReadings", "Chart.Start", "Chart.Config.ChannelSelection", "Chart.Config", "Chart.Config.DataToPlot", "Chart.Config.SamplingRate.Units", "Chart.Config.ClearBuffer", "Ratio.Mode", "InternalRef.Frequency.Increment": Mouse Leave {
            n51 = event-data() -> ()  [unwired: 1 in, 1 out]
            n52 = call "VI Server_SetCursor_ARROW.vi"("error in"=w109, "VI Server.RefsCluster"=w108) -> ("error out"=w107:errorcluster)  [unwired: 8 in, 1 out]
          }
          event "UDP.IP.Address": Value Change {
            n53 = event-data() -> ("NewVal"=w111:string)  [unwired: 1 in]
            n54 = call "NAI8810A_Accessor_UDP_IP_Address_Ref.vi"() -> ("UDP.IP.Address"=w112:refnum<notifier>)  [unwired: 6 in]
            n55 = String To IP(1:w111) -> (0:w110:u32)
            n56 = Send Notification(notification=w110, notifier=w112, error in (no error)=w114) -> (error out=w113:errorcluster)  [unwired: 1 out]
          }
          event "UDP.LocalPort.Write": Value Change {
            n57 = event-data() -> ("NewVal"=w115:u16)  [unwired: 1 in]
            n58 = call "NAI8810A_Accessor_UDP_LocalPort_Write_Ref.vi"() -> ("UDP.LocalPort.Write"=w116:refnum<notifier>)  [unwired: 6 in]
            n59 = Send Notification(notification=w115, notifier=w116, error in (no error)=w118) -> (error out=w117:errorcluster)  [unwired: 1 out]
          }
          event "UDP.Port.RT": Value Change {
            n60 = event-data() -> ("NewVal"=w120:u16)  [unwired: 1 in]
            n61 = call "NAI8810A_Accessor_UDP_Port_Read_Ref.vi"() -> ("UDP.Port.Read"=w119:refnum<notifier>)  [unwired: 6 in]
            n62 = Send Notification(notification=w120, notifier=w119, error in (no error)=w122) -> (error out=w121:errorcluster)  [unwired: 1 out]
          }
          event "UDP.Port.BC": Value Change {
            n63 = event-data() -> ("NewVal"=w124:u16)  [unwired: 1 in]
            n64 = call "NAI8810A_Accessor_UDP_Port_Receiver_Ref.vi"() -> ("UDP.Port.Receiver"=w123:refnum<notifier>)  [unwired: 6 in]
            n65 = Send Notification(notification=w124, notifier=w123, error in (no error)=w126) -> (error out=w125:errorcluster)  [unwired: 1 out]
          }
          event "UDP.Responce.String.Monitor": Value Change {
            n66 = event-data() -> ("NewVal"=w129:bool)  [unwired: 1 in]
            n67 = call "NAI8810A_Accessor_UDP_Responce_String_Monitor_Ref.vi"() -> ("UDP.ExecEng.Command.String.Monitor"=w128:refnum<notifier>)  [unwired: 6 in]
            n68 = Send Notification(notification=w129, notifier=w128, error in (no error)=w130) -> (error out=w127:errorcluster)  [unwired: 1 out]
          }
          event "UDP.Test.String1.Send": Value Change {
            n69 = event-data() -> ()  [unwired: 1 in, 1 out]
            n70 = call-poly "VI Server_GetControl_Value_Ref.vi"("DataType"="", "Control.Label"="UDP.Test.String1", "error in"=w142, "SingleInstance"=TRUE, "VI Server.RefsCluster"=w140) -> ("error out"=w135:errorcluster, "Value"=w131:string)  [unwired: 3 in, 2 out]
            n71 = Format Into String(format string="%s\\r\\n", error in=w135, w131) -> (resulting string=w133:string, error out=w134:errorcluster)  [unwired: 1 in]
            n72 = call "NAI8810A_Accessor_TCP_IP_WriteQ_Ref.vi"() -> ("TCP/IP.Write.Q"=w136:refnum<queue>)  [unwired: 6 in]
            n73 = Enqueue Element(queue=w136, element=w133, error in (no error)=w134) -> (error out=w141:errorcluster)  [unwired: 1 in, 2 out]
          }
          event "UDP.Test.String2.Send": Value Change {
            n74 = event-data() -> ()  [unwired: 1 in, 1 out]
            n75 = call-poly "VI Server_GetControl_Value_Ref.vi"("DataType"="", "Control.Label"="UDP.Test.String2", "error in"=w154, "SingleInstance"=TRUE, "VI Server.RefsCluster"=w152) -> ("error out"=w147:errorcluster, "Value"=w143:string)  [unwired: 3 in, 2 out]
            n76 = Format Into String(format string="%s\\r\\n", error in=w147, w143) -> (resulting string=w145:string, error out=w146:errorcluster)  [unwired: 1 in]
            n77 = call "NAI8810A_Accessor_TCP_IP_WriteQ_Ref.vi"() -> ("TCP/IP.Write.Q"=w148:refnum<queue>)  [unwired: 6 in]
            n78 = Enqueue Element(queue=w148, element=w145, error in (no error)=w146) -> (error out=w153:errorcluster)  [unwired: 1 in, 2 out]
          }
          event "MonitorCommandExecution": Value Change {
            n79 = event-data() -> ("NewVal"=w157:bool)  [unwired: 1 in]
            n80 = call "NAI8810A_Accessor_TCP_IP_MonitorReadString_Ref.vi"() -> ("TCP/IP.MonitorReadString"=w156:refnum<notifier>)  [unwired: 6 in]
            n81 = Send Notification(notification=w157, notifier=w156, error in (no error)=w158) -> (error out=w155:errorcluster)  [unwired: 1 out]
          }
          event "Tab.Ch1.Ch2", "Tab.Ch1.DualCh", "Tab.Ch1.IntRef", "Tab.Ch1.SetUp", "Tab.Ch1.Help", "UDP.Setup", "Tab.Ch2.Help", "Tab.Ch2.SetUp", "Tab.Ch2.IntRef", "Tab.Ch2.DualCh", "Tab.Ch2.Ch1", "Tab.Ch2.Ch2", "Tab.Ch1-2.SetUp", "Tab.Ch1-2.IntRef", "Tab.Ch1-2.Ch2", "Tab.Ch1-2.Ch1", "Tab.Ch1-2.Ch1-2", "Tab.IntRef.SetUp", "Tab.IntRef.Ch1-2", "Tab.IntRef.Ch2", "Tab.IntRef.Ch1", "Tab.IntRef.IntRef", "TCP/IP.Setup": Value Change {
            n82 = event-data() -> ("CtlRef"=w162:refnum<vi>)  [unwired: 1 in]
            n83 = control-ref of="Tab.Main"() -> (w161:refnum<vi>)
            n84 = call "NAI8810A_TabSwitch.vi"("CtlRef"=w162, "Tab.Main.Ref"=w161, "error in"=w160, "VI Server Cluster"=w159) -> ("error out"=w163:errorcluster)  [unwired: 7 in]
          }
          event "Ch1-2.Ch1.Internal/External.Ref", "Ch1.Internal/External.Ref": Value Change {
            # "ON = EXT; OFF =INT"
            n85 = event-data() -> ("NewVal"=w176:bool)  [unwired: 1 in]
            n86 = call "NAI8810A_Accessor_ActiveChannel_Ref.vi"() -> ("ActiveChannel"=w171:refnum<notifier>)  [unwired: 6 in]
            n87 = Send Notification(notification=u8 1, notifier=w171, error in (no error)=w168) -> (error out=w169:errorcluster)  [unwired: 1 out]
            n88 = call "NAI8810A_Accessor_Command_Value1_Ref.vi"() -> ("Command.Value.1"=w173:refnum<notifier>)  [unwired: 6 in]
            n89 = Select(t="EXT", s=w176, f="INT") -> (s? t:f=w172:string)
            n90 = call "NAI8810A_Accessor_Command_Ref.vi"() -> ("Command"=w165:refnum<queue>)  [unwired: 6 in]
            n91 = Send Notification(notification=w172, notifier=w173, error in (no error)=w169) -> (error out=w167:errorcluster)  [unwired: 1 out]
            n92 = Flush Queue(queue=w165, error in (no error)=w167) -> (queue out=w164:refnum<queue>, error out=w166:errorcluster)  [unwired: 1 out]
            n93 = Enqueue Element(queue=w164, element=NAI8810A_Command."Reference Mode", error in (no error)=w166) -> (error out=w178:errorcluster)  [unwired: 1 in, 2 out]
          }
          event "Ch1-2.Ch2.Internal/External.Ref", "Ch2.Internal/External.Ref": Value Change {
            # "ON = EXT; OFF =INT"
            n94 = event-data() -> ("NewVal"=w191:bool)  [unwired: 1 in]
            n95 = call "NAI8810A_Accessor_ActiveChannel_Ref.vi"() -> ("ActiveChannel"=w186:refnum<notifier>)  [unwired: 6 in]
            n96 = Send Notification(notification=u8 2, notifier=w186, error in (no error)=w183) -> (error out=w184:errorcluster)  [unwired: 1 out]
            n97 = call "NAI8810A_Accessor_Command_Value1_Ref.vi"() -> ("Command.Value.1"=w188:refnum<notifier>)  [unwired: 6 in]
            n98 = Select(t="EXT", s=w191, f="INT") -> (s? t:f=w187:string)
            n99 = call "NAI8810A_Accessor_Command_Ref.vi"() -> ("Command"=w180:refnum<queue>)  [unwired: 6 in]
            n100 = Send Notification(notification=w187, notifier=w188, error in (no error)=w184) -> (error out=w182:errorcluster)  [unwired: 1 out]
            n101 = Flush Queue(queue=w180, error in (no error)=w182) -> (queue out=w179:refnum<queue>, error out=w181:errorcluster)  [unwired: 1 out]
            n102 = Enqueue Element(queue=w179, element=NAI8810A_Command."Reference Mode", error in (no error)=w181) -> (error out=w193:errorcluster)  [unwired: 1 in, 2 out]
          }
          event "Ch1.SYN/RSL": Value Change {
            # "ON = SYN; OFF =RES"
            n103 = event-data() -> ("NewVal"=w203:bool)  [unwired: 1 in]
            n104 = call "NAI8810A_Accessor_ActiveChannel_Ref.vi"() -> ("ActiveChannel"=w201:refnum<notifier>)  [unwired: 6 in]
            n105 = Send Notification(notification=u8 1, notifier=w201, error in (no error)=w198) -> (error out=w199:errorcluster)  [unwired: 1 out]
            n106 = call "NAI8810A_Accessor_Command_Value1_Ref.vi"() -> ("Command.Value.1"=w206:refnum<notifier>)  [unwired: 6 in]
            n107 = Select(t="SYN", s=w203, f="RSL") -> (s? t:f=w205:string)
            n108 = Send Notification(notification=w205, notifier=w206, error in (no error)=w199) -> (error out=w195:errorcluster)  [unwired: 1 out]
            n109 = call "NAI8810A_Accessor_Command_Ref.vi"() -> ("Command"=w197:refnum<queue>)  [unwired: 6 in]
            n110 = Flush Queue(queue=w197, error in (no error)=w195) -> (queue out=w196:refnum<queue>, error out=w194:errorcluster)  [unwired: 1 out]
            n111 = Enqueue Element(queue=w196, element=NAI8810A_Command."Signal Mode", error in (no error)=w194) -> (error out=w204:errorcluster)  [unwired: 1 in, 2 out]
          }
          event "Ch2.SYN/RSL", "Ch1-2.Ch2.SYN/RSL": Value Change {
            # "ON = SYN; OFF =RES"
            n112 = event-data() -> ("NewVal"=w218:bool)  [unwired: 1 in]
            n113 = call "NAI8810A_Accessor_ActiveChannel_Ref.vi"() -> ("ActiveChannel"=w216:refnum<notifier>)  [unwired: 6 in]
            n114 = Send Notification(notification=u8 1, notifier=w216, error in (no error)=w213) -> (error out=w214:errorcluster)  [unwired: 1 out]
            n115 = call "NAI8810A_Accessor_Command_Value1_Ref.vi"() -> ("Command.Value.1"=w221:refnum<notifier>)  [unwired: 6 in]
            n116 = Select(t="SYN", s=w218, f="RES") -> (s? t:f=w220:string)
            n117 = Send Notification(notification=w220, notifier=w221, error in (no error)=w214) -> (error out=w210:errorcluster)  [unwired: 1 out]
            n118 = call "NAI8810A_Accessor_Command_Ref.vi"() -> ("Command"=w212:refnum<queue>)  [unwired: 6 in]
            n119 = Flush Queue(queue=w212, error in (no error)=w210) -> (queue out=w211:refnum<queue>, error out=w209:errorcluster)  [unwired: 1 out]
            n120 = Enqueue Element(queue=w211, element=NAI8810A_Command."Signal Mode", error in (no error)=w209) -> (error out=w219:errorcluster)  [unwired: 1 in, 2 out]
          }
          event "Ch1.Ratio", "Ch2.Ratio", "Ch1-2.Ratio", "InternalRef.Ratio": Value Change {
            n121 = event-data() -> ()  [unwired: 1 in, 1 out]
            n122 = call "NAI8810A_Ratio.vi"("error in"=w225) -> ("error out"=w224:errorcluster)  [unwired: 10 in]
          }
          event "Ratio.Mode": Value Change {
            n123 = event-data() -> ()  [unwired: 1 in, 1 out]
            n124 = call "NAI8810A_Ratio_Mode.vi"("error in"=w228, "VI Server.RefsCluster"=w226) -> ("error out"=w227:errorcluster)  [unwired: 8 in, 1 out]
          }
          event "Ratio.Value": Value Change {
            n125 = event-data() -> ()  [unwired: 1 in, 1 out]
            n126 = call "NAI8810A_Ratio_Value.vi"("error in"=w231, "VI Server.RefsCluster"=w229) -> ("error out"=w230:errorcluster)  [unwired: 8 in, 1 out]
          }
          event "Ch1.Input.Front/Rear", "Ch1-2.Input.Front/Rear", "Ch2.Input.Front/Rear", "InternalRef.Input.Front/Rear": Value Change {
            # "ON = BACK; OFF =FRONT"
            n127 = event-data() -> ("NewVal"=w238:bool)  [unwired: 1 in]
            n128 = call "NAI8810A_Accessor_Command_Value1_Ref.vi"() -> ("Command.Value.1"=w242:refnum<notifier>)  [unwired: 6 in]
            n129 = Select(t="FRONT", s=w238, f="BACK") -> (s? t:f=w241:string)
            n130 = Send Notification(notification=w241, notifier=w242, error in (no error)=w239) -> (error out=w233:errorcluster)  [unwired: 1 out]
            n131 = call "NAI8810A_Accessor_Command_Ref.vi"() -> ("Command"=w235:refnum<queue>)  [unwired: 6 in]
            n132 = Flush Queue(queue=w235, error in (no error)=w233) -> (queue out=w234:refnum<queue>, error out=w232:errorcluster)  [unwired: 1 out]
            n133 = Enqueue Element(queue=w234, element=NAI8810A_Command."Channel 1 Input Connector", error in (no error)=w232) -> (error out=w240:errorcluster)  [unwired: 1 in, 2 out]
          }
          event "Ch1.Local/Remote", "Ch2.Local/Remote", "Ch1-2.Local/Remote", "InternalRef.Local/Remote": Value Change {
            n134 = event-data() -> ("NewVal"=w250:bool)  [unwired: 1 in]
            n135 = call "NAI8810A_Accessor_Command_Value1_Ref.vi"() -> ("Command.Value.1"=w254:refnum<notifier>)  [unwired: 6 in]
            n136 = Select(t="LOCKOUT", s=w250, f="LOCAL") -> (s? t:f=w253:string)
            n137 = Send Notification(notification=w253, notifier=w254, error in (no error)=w251) -> (error out=w247:errorcluster)  [unwired: 1 out]
            n138 = call "NAI8810A_Accessor_Command_Ref.vi"() -> ("Command"=w245:refnum<queue>)  [unwired: 6 in]
            n139 = Flush Queue(queue=w245, error in (no error)=w247) -> (queue out=w244:refnum<queue>, error out=w246:errorcluster)  [unwired: 1 out]
            n140 = Enqueue Element(queue=w244, element=NAI8810A_Command."LOCAL/REMOTE", error in (no error)=w246) -> (error out=w252:errorcluster)  [unwired: 1 in, 2 out]
          }
          event "Ch1.Hold", "Ch2.Hold", "Ch1-2.Ch1.Hold", "Ch1-2.Ch2.Hold": Value Change {
            # "API<chan><b>UPDATE<b><LATCH|TRACK><cr><lf>"
            # "ON = TRACK; OFF =LATCH"
            n141 = event-data() -> ("CtlRef"=w256:refnum<vi>)  [unwired: 1 in]
            n142 = call "NAI8810A_Hold.vi"("CtlRef"=w256, "error in (no error)"=w258, "VI Server.RefsCluster"=w257) -> ("error out"=w259:errorcluster)  [unwired: 7 in, 1 out]
          }
          event "Ch1.Ave.AnglesReadings", "Ch2.Ave.AnglesReadings", "Ch1-2.Ch1.Ave.AnglesReadings", "Ch1-2.Ch2.Ave.AnglesReadings": Value Change {
            n143 = event-data() -> ()  [unwired: 1 in, 1 out]
            n144 = call "NAI8810A_AverageAngleReadings.vi"("error in"=w260) -> ("error out"=w261:errorcluster)  [unwired: 10 in]
          }
          event "Ch1.AverageAnglesReadings", "Ch2.AverageAnglesReadings": Value Change {
            n145 = event-data() -> ("CtlRef"=w263:refnum<vi>)  [unwired: 1 in]
            n146 = call "NAI8810A_AveragingAngleReadings.vi"("CtlRef"=w263, "error in (no error)"=w264) -> ("error out"=w262:errorcluster)  [unwired: 9 in]
          }
          event "Ch1.AveragingInterval", "Ch2.AveragingInterval": Value Change {
            n147 = event-data() -> ("CtlRef"=w265:refnum<vi>)  [unwired: 1 in]
            n148 = call "NAI8810A_AveragingAngleReadingsInterval.vi"("CtlRef"=w265, "error in (no error)"=w267) -> ("error out"=w266:errorcluster)  [unwired: 9 in]
          }
          event "AveAnglesReadings.DONE", "TestAnglesReadings.DONE", "Ratio.DONE", "Chart.DONE", "Setup.DONE", "TCP/IP.DONE": Value Change {
            n149 = event-data() -> ()  [unwired: 1 in, 1 out]
            n150 = call "NAI8810A_AverageAngleReadings_DONE.vi"("error in"=w269) -> ("error out"=w268:errorcluster)  [unwired: 10 in]
          }
          event "GraphConfig.DONE": Value Change {
            n151 = event-data() -> ()  [unwired: 1 in, 1 out]
            n152 = call "NAI8810A_Accessor_Tab_Main_Ref.vi"() -> ("Tab.Main.Ref"=w275:refnum<notifier>)  [unwired: 6 in]
            n153 = Get Notifier Status(notifier=w275, error in (no error)=w272) -> (current notification=w274:refnum<vi>, error out=w273:errorcluster)  [unwired: 3 out]
            n154 = property class="TabCtl (strict)"(reference=w274, error in=w273, "Value"=T1."Graph") -> (error out=w271:errorcluster)  [unwired: 1 out]
          }
          event "Ch1.TestAngleReadings", "Ch2.TestAngleReadings", "Ch1-2.Ch2.TestAngleReadings", "Ch1-2.Ch1.TestAngleReadings": Value Change {
            n155 = event-data() -> ()  [unwired: 1 in, 1 out]
            n156 = call "NAI8810A_Accessor_Tab_Main_Ref.vi"() -> ("Tab.Main.Ref"=w281:refnum<notifier>)  [unwired: 6 in]
            n157 = Get Notifier Status(notifier=w281, error in (no error)=w277) -> (current notification=w280:refnum<vi>, error out=w279:errorcluster)  [unwired: 3 out]
            n158 = property class="TabCtl (strict)"(reference=w280, error in=w279, "Value"=T7."TestAngle") -> (error out=w278:errorcluster)  [unwired: 1 out]
          }
          event "Ch1.TestAngleReading.ENBL", "Ch2.TestAngleReading.ENBL": Value Change {
            n159 = event-data() -> ("CtlRef"=w282:refnum<vi>)  [unwired: 1 in]
            n160 = call "NAI8810A_TestAngleReadings_Enable.vi"("CtlRef"=w282, "error in (no error)"=w285, "VI Server.RefsCluster"=w283) -> ("error out"=w284:errorcluster)  [unwired: 7 in, 1 out]
          }
          event "Ch1.TestAngleReading.Comparision.Mode", "Ch2.TestAngleReading.Comparision.Mode": Value Change {
            n161 = event-data() -> ("CtlRef"=w292:refnum<vi>)  [unwired: 1 in]
            n162 = property class="Bool (strict)"(reference=w292, error in=w293) -> (error out=w291:errorcluster, "Label.Text"=w294:string)  [unwired: 1 out]
            n163 = case shown="\"Ch2.TestAngleReading.Comparision.Mode\"" w294 {
              tunnel: [u8 1 ("notification") u8 2 ("notification")] -> w288
              frame "Ch1.TestAngleReading.Comparision.Mode", Default {
              }
              frame "Ch2.TestAngleReading.Comparision.Mode" {
              }
            }
            n164 = call "NAI8810A_Accessor_ActiveChannel_Ref.vi"() -> ("ActiveChannel"=w287:refnum<notifier>)  [unwired: 6 in]
            n165 = Send Notification(notification=w288, notifier=w287, error in (no error)=w291) -> (error out=w290:errorcluster)  [unwired: 1 out]
            n166 = call "NAI8810A_TestAngleReadings_ComparisionMode.vi"("error in (no error)"=w290, "VI Server.RefsCluster"=w286) -> ("error out"=w289:errorcluster)  [unwired: 8 in, 1 out]
          }
          event "Ch1.TestAngleReading.Limit.HI", "Ch2.TestAngleReading.Limit.HI": Value Change {
            n167 = event-data() -> ("CtlRef"=w303:refnum<vi>)  [unwired: 1 in]
            n168 = property class="DigNum (strict)"(reference=w303, error in=w304) -> (error out=w302:errorcluster, "Label.Text"=w305:string)  [unwired: 1 out]
            n169 = case shown="\"Ch2.TestAngleReading.Limit.HI\"" w305 {
              tunnel: [u8 1 ("notification") u8 2 ("notification")] -> w301
              frame "Ch1.TestAngleReading.Limit.HI", Default {
              }
              frame "Ch2.TestAngleReading.Limit.HI" {
              }
            }
            n170 = call "NAI8810A_Accessor_ActiveChannel_Ref.vi"() -> ("ActiveChannel"=w300:refnum<notifier>)  [unwired: 6 in]
            n171 = Send Notification(notification=w301, notifier=w300, error in (no error)=w302) -> (error out=w299:errorcluster)  [unwired: 1 out]
            n172 = call "NAI8810A_TestAngleReadings_LimitHI.vi"("error in (no error)"=w299, "VI Server.RefsCluster"=w297) -> ("error out"=w298:errorcluster)  [unwired: 8 in, 1 out]
          }
          event "Ch1.TestAngleReading.Limit.LO", "Ch2.TestAngleReading.Limit.LO": Value Change {
            n173 = event-data() -> ("CtlRef"=w314:refnum<vi>)  [unwired: 1 in]
            n174 = property class="DigNum (strict)"(reference=w314, error in=w315) -> (error out=w313:errorcluster, "Label.Text"=w316:string)  [unwired: 1 out]
            n175 = case shown="\"Ch2.TestAngleReading.Limit.LO\"" w316 {
              tunnel: [u8 1 ("notification") u8 2 ("notification")] -> w312
              frame "Ch1.TestAngleReading.Limit.LO", Default {
              }
              frame "Ch2.TestAngleReading.Limit.LO" {
              }
            }
            n176 = call "NAI8810A_Accessor_ActiveChannel_Ref.vi"() -> ("ActiveChannel"=w311:refnum<notifier>)  [unwired: 6 in]
            n177 = Send Notification(notification=w312, notifier=w311, error in (no error)=w313) -> (error out=w310:errorcluster)  [unwired: 1 out]
            n178 = call "NAI8810A_TestAngleReadings_LimitLO.vi"("error in (no error)"=w310, "VI Server.RefsCluster"=w308) -> ("error out"=w309:errorcluster)  [unwired: 8 in, 1 out]
          }
          event "Ch1.TestAngleReading.Step", "Ch2.TestAngleReading.Step": Value Change {
            n179 = event-data() -> ("CtlRef"=w325:refnum<vi>)  [unwired: 1 in]
            n180 = property class="DigNum (strict)"(reference=w325, error in=w326) -> (error out=w324:errorcluster, "Label.Text"=w327:string)  [unwired: 1 out]
            n181 = case shown="\"Ch2.TestAngleReading.Step\"" w327 {
              tunnel: [u8 1 ("notification") u8 2 ("notification")] -> w323
              frame "Ch1.TestAngleReading.Step", Default {
              }
              frame "Ch2.TestAngleReading.Step" {
              }
            }
            n182 = call "NAI8810A_Accessor_ActiveChannel_Ref.vi"() -> ("ActiveChannel"=w322:refnum<notifier>)  [unwired: 6 in]
            n183 = Send Notification(notification=w323, notifier=w322, error in (no error)=w324) -> (error out=w321:errorcluster)  [unwired: 1 out]
            n184 = call "NAI8810A_TestAngleReadings_Step.vi"("error in (no error)"=w321, "VI Server.RefsCluster"=w319) -> ("error out"=w320:errorcluster)  [unwired: 8 in, 1 out]
          }
          event "InternalRef.26V", "InternalRef.115V": Value Change {
            n185 = event-data() -> ("CtlRef"=w330:refnum<vi>)  [unwired: 1 in]
            n186 = call "NAI8810A_InternalReferenceVoltagePresets_Manage.vi"("CtlRef"=w330, "error in"=w333, "VI Server.RefsCluster"=w331) -> ("error out"=w332:errorcluster)  [unwired: 7 in, 1 out]
          }
          event "InternalRef.Voltage": Value Change {
            n187 = event-data() -> ()  [unwired: 1 in, 1 out]
            n188 = call "NAI8810A_InternalReferenceGenerator_Voltage_SET.vi"("error in"=w335, "VI Server.RefsCluster"=w334) -> ("error out"=w336:errorcluster)  [unwired: 8 in, 1 out]
          }
          event "InternalRef.Frequency": Value Change {
            n189 = event-data() -> ()  [unwired: 1 in, 1 out]
            n190 = call "NAI8810A_InternalReferenceGenerator_Frequency_SET.vi"("error in"=w339, "VI Server.RefsCluster"=w338) -> ("error out"=w337:errorcluster)  [unwired: 8 in, 1 out]
          }
          event "InternalRef.Frequency.Increment": Value Change {
            n191 = event-data() -> ()  [unwired: 1 in, 1 out]
            n192 = call <vilib>:"Intialize Keyboard.vi"("error in (no error)"=w343) -> ("error out"=w342:errorcluster, "device ID"=w340:refnum<k1>)  [unwired: 9 in]
            n193 = call-poly <vilib>:"Close Input Device.vi"("error in (no error)"=w342, "device ID"=w340) -> ("error out"=w341:errorcluster)  [unwired: 8 in]
          }
          event "InternalRef.Signal.Out": Value Change {
            n194 = event-data() -> ()  [unwired: 1 in, 1 out]
            n195 = call "NAI8810A_InternalReferenceGenerator_OutputState_SET.vi"("error in"=w346, "VI Server.RefsCluster"=w345) -> ("error out"=w344:errorcluster)  [unwired: 8 in, 1 out]
          }
          event Value Change {
            n196 = event-data() -> ("NewVal"=w347:T2)  [unwired: 1 in]
            n197 = call "NAI8810A_ShowAngleDifference.vi"("NewVal"=w347, "error in (no error)"=w350, "VI Server.RefsCluster"=w348) -> ("error out"=w349:errorcluster)  [unwired: 8 in]
          }
          event "UpdateTime.Degrees": Value Change {
            n198 = event-data() -> ("NewVal"=w352:u32)  [unwired: 1 in]
            n199 = call "NAI8810A_Accessor_UpdateTime_UpdateDegrees_Ref.vi"() -> ("UpdateTime.Degrees"=w351:refnum<notifier>)  [unwired: 6 in]
            n200 = Send Notification(notification=w352, notifier=w351, error in (no error)=w354) -> (error out=w353:errorcluster)  [unwired: 1 out]
          }
          event "UpdateTime.Ref.Parameters": Value Change {
            n201 = event-data() -> ("NewVal"=w356:u32)  [unwired: 1 in]
            n202 = call "NAI8810A_Accessor_UpdateTime_Ref_Parameters_Ref.vi"() -> ("UpdateTime.Ref.Parameters"=w355:refnum<notifier>)  [unwired: 6 in]
            n203 = Send Notification(notification=w356, notifier=w355, error in (no error)=w358) -> (error out=w357:errorcluster)  [unwired: 1 out]
          }
          event "AngleDisplay.Format": Value Change {
            n204 = event-data() -> ()  [unwired: 1 in, 1 out]
            n205 = call "VI Server_Get Text Ring Selection.vi"("Label"="AngleDisplay.Format", "error in"=w371, "Single Instance (T)"=TRUE, "VI Server Cluster"=w370) -> ("error out"=w365:errorcluster, "Selection"=w364:string)  [unwired: 2 in, 4 out]
            n206 = call "NAI8810A_Accessor_Command_Value1_Ref.vi"() -> ("Command.Value.1"=w368:refnum<notifier>)  [unwired: 6 in]
            n207 = call "NAI8810A_Accessor_Command_Ref.vi"() -> ("Command"=w360:refnum<queue>)  [unwired: 6 in]
            n208 = Send Notification(notification=w364, notifier=w368, error in (no error)=w365) -> (error out=w362:errorcluster)  [unwired: 1 out]
            n209 = Flush Queue(queue=w360, error in (no error)=w362) -> (queue out=w359:refnum<queue>, error out=w361:errorcluster)  [unwired: 1 out]
            n210 = Enqueue Element(queue=w359, element=NAI8810A_Command."AngleDisplay.Format", error in (no error)=w361) -> (error out=w363:errorcluster)  [unwired: 1 in, 2 out]
          }
          event "AngleResolution": Value Change {
            n211 = event-data() -> ()  [unwired: 1 in, 1 out]
            n212 = call "VI Server_Get Text Ring Selection.vi"("Label"="AngleResolution", "error in"=w384, "Single Instance (T)"=TRUE, "VI Server Cluster"=w383) -> ("error out"=w378:errorcluster, "Selection"=w377:string)  [unwired: 2 in, 4 out]
            n213 = call "NAI8810A_Accessor_Command_Value1_Ref.vi"() -> ("Command.Value.1"=w381:refnum<notifier>)  [unwired: 6 in]
            n214 = call "NAI8810A_Accessor_Command_Ref.vi"() -> ("Command"=w373:refnum<queue>)  [unwired: 6 in]
            n215 = Send Notification(notification=w377, notifier=w381, error in (no error)=w378) -> (error out=w375:errorcluster)  [unwired: 1 out]
            n216 = Flush Queue(queue=w373, error in (no error)=w375) -> (queue out=w372:refnum<queue>, error out=w374:errorcluster)  [unwired: 1 out]
            n217 = Enqueue Element(queue=w372, element=NAI8810A_Command."Angles.Resolution", error in (no error)=w374) -> (error out=w376:errorcluster)  [unwired: 1 in, 2 out]
          }
          event "Ch1.AutoBandwidth", "Ch2.AutoBandwidth": Value Change {
            n218 = event-data() -> ("CtlRef"=w385:refnum<vi>)  [unwired: 1 in]
            n219 = call "NAI8810A_Bandwidth_AUTO.vi"("CtlRef"=w385, "error in (no error)"=w387, "VI Server Cluster"=w386) -> ("error out"=w388:errorcluster)  [unwired: 7 in, 1 out]
          }
          event "Ch1.Bandwidth.Value", "Ch2.Bandwidth.Value": Value Change {
            n220 = event-data() -> ("CtlRef"=w389:refnum<vi>)  [unwired: 1 in]
            n221 = call "NAI8810A_Bandwidth_SET.vi"("CtlRef"=w389, "error in (no error)"=w392, "VI Server Cluster"=w391) -> ("error out"=w390:errorcluster)  [unwired: 7 in, 1 out]
          }
          event "Ch1.Graph", "Ch2.Graph", "Ch1-2.Graph", "InternalRef.Graph": Value Change {
            n222 = event-data() -> ()  [unwired: 1 in, 1 out]
            n223 = call "NAI8810A_Accessor_Tab_Main_Ref.vi"() -> ("Tab.Main.Ref"=w396:refnum<notifier>)  [unwired: 6 in]
            n224 = Get Notifier Status(notifier=w396, error in (no error)=w395) -> (current notification=w397:refnum<vi>, error out=w398:errorcluster)  [unwired: 3 out]
            n225 = property class="TabCtl (strict)"(reference=w397, error in=w398, "Value"=T8."Graph") -> (error out=w394:errorcluster)  [unwired: 1 out]
          }
          event "Chart.Start": Value Change {
            n226 = event-data() -> ("NewVal"=w399:bool)  [unwired: 1 in]
            n227 = call "NAI8810A_Graph_Start_Stop.vi"("Chart.Start"=w399, "error in (no error)"=w402, "VI Server Cluster"=w400) -> ("error out"=w401:errorcluster)  [unwired: 7 in, 1 out]
          }
          event "Chart.Config.ClearBuffer": Value Change {
            n228 = event-data() -> ()  [unwired: 1 in, 1 out]
            n229 = call "NAI8810A_Accessor_Command_Ref.vi"() -> ("Command"=w404:refnum<queue>)  [unwired: 6 in]
            n230 = Flush Queue(queue=w404, error in (no error)=w405) -> (queue out=w403:refnum<queue>, error out=w406:errorcluster)  [unwired: 1 out]
            n231 = Enqueue Element(queue=w403, element=NAI8810A_Command."Clear Buffer", error in (no error)=w406) -> (error out=w407:errorcluster)  [unwired: 1 in, 2 out]
          }
          event "Chart.Config": Value Change {
            n232 = event-data() -> ()  [unwired: 1 in, 1 out]
            n233 = call "NAI8810A_Accessor_Tab_Main_Ref.vi"() -> ("Tab.Main.Ref"=w414:refnum<notifier>)  [unwired: 6 in]
            n234 = Get Notifier Status(notifier=w414, error in (no error)=w411) -> (current notification=w413:refnum<vi>, error out=w412:errorcluster)  [unwired: 3 out]
            n235 = property class="TabCtl (strict)"(reference=w413, error in=w412, "Value"=T1."Graph.Config") -> (error out=w410:errorcluster)  [unwired: 1 out]
          }
          event "Chart.Config.ChannelSelection": Value Change {
            n236 = event-data() -> ()  [unwired: 1 in, 1 out]
            n237 = call "NA8810A_Graph_Configuration_ChannelSelection.vi"("error in (no error)"=w417, "VI Server Cluster"=w416) -> ("error out"=w415:errorcluster)  [unwired: 8 in, 1 out]
          }
          event "Chart.Config.DataToPlot": Value Change {
            n238 = event-data() -> ()  [unwired: 1 in, 1 out]
            n239 = call "NAI8810A_Graph_Configuration_DataToPlot.vi"("error in (no error)"=w420, "VI Server Cluster"=w419) -> ("error out"=w418:errorcluster)  [unwired: 8 in, 1 out]
          }
          event "Chart.Config.DataToPlot.Step": Value Change {
            n240 = event-data() -> ()  [unwired: 1 in, 1 out]
            n241 = call "NA8810A_Graph_Config_AngleStep.vi"("error in (no error)"=w423, "VI Server Cluster"=w422) -> ("error out"=w421:errorcluster)  [unwired: 8 in, 1 out]
          }
          event "Chart.Config.SamplingRate": Value Change {
            n242 = event-data() -> ()  [unwired: 1 in, 1 out]
            n243 = call "NAI8810A_Graph_Configuration_SamplingRate.vi"("error in (no error)"=w424, "VI Server Cluster"=w426) -> ("error out"=w425:errorcluster)  [unwired: 8 in, 1 out]
          }
          event "Chart.Config.SamplingRate.Units": Value Change {
            n244 = event-data() -> ()  [unwired: 1 in, 1 out]
            n245 = call "VI Server_CycleEventBySignalingValue.vi"("Label"="Chart.Config.SamplingRate", "error in"=w430, "VI Server.RefsCluster"=w428) -> ("error out"=w429:errorcluster)  [unwired: 7 in, 1 out]
          }
        }
        n246 = call "NAI8810A_Accessor_EXIT_Ref.vi"() -> ("EXIT"=w41:refnum<notifier>)  [unwired: 6 in]
        n247 = call "StopOnErrorOrCommand.vi"("STOP"=w41, "error in (no error)"=w43) -> ("error out"=w44:errorcluster, "STOP"=w42:bool)  [unwired: 8 in]
      }
      n248 = call "NAI_UDP_MAIN.vi"("error in (no error)"=w27, "VI Server.RefsCluster"=w28) -> ("error out"=w33:errorcluster)  [unwired: 9 in]
      n249 = call "NAI8810A_CommandsProcessor_MAIN.vi"("error in"=w27, "VI Server.RefsCluster"=w28) -> ("error out"=w30:errorcluster)  [unwired: 8 in, 1 out]
      n250 = call "NAI8810A_CommandsGenerator_MAIN.vi"("error in"=w27) -> ("error out"=w29:errorcluster)  [unwired: 10 in]
      n251 = call "NAI8810A_TCP_IP_Interface_MAIN.vi"("error in"=w27, "VI Server.RefsCluster"=w28) -> ("error out"=w26:errorcluster)  [unwired: 9 in]
      n252 = Build Array(w26, w29, w30, w33) -> (w32:errorcluster[])
      n253 = call "Merge Errors II.vi"("error array in"=w32, "error in 1 (no error)"=w35) -> ("error out.DUP"=w34:errorcluster)  [unwired: 4 in, 1 out]
    }
    frame Error {
    }
  }
  n254 = call "VI Server_CloseRefs.vi"("error in"=w20, "VI Server.RefsCluster"=w18) -> ("error out"=w19:errorcluster)  [unwired: 9 in]
  n255 = call "NAI8810A_Synch_CLOSE.vi"("error in"=w19) -> ("error out"=w6:errorcluster)  [unwired: 10 in]
  n256 = Current VI's Path() -> (path=w4:path)
  n257 = call "Close Window If in EXE mode.vi"("TopLevelVI Path"=w4, "error in"=w6) -> ("error out"=→"error out":errorcluster)  [unwired: 9 in]
